vi "Find Target Actor.vi"(5 "Target":refnum<vi>, 7 "App Inst":refnum<vi>, 8 "error in (no error)":errorcluster, 11 "Message Path":path) -> (0 "error out":errorcluster, 3 "Targeted Actor":path)   [LabVIEW 2020, in "Message Rescripter.lvlib"]
uses:
  Message Rescripter.lvlib
  <vilib>/Utility/traverseref.llb/TRef TravTarget.ctl
  <vilib>/Utility/traverseref.llb/VI Scripting - Traverse.lvlib
  <vilib>/Utility/Data Type/NI_Data Type.lvlib
  <vilib>/ErrorRing/Error Ring.xnode
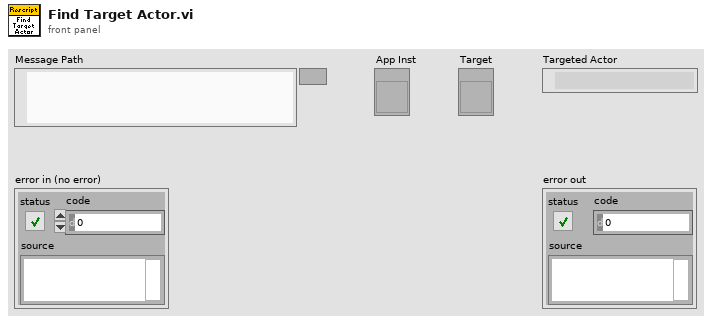
[diagram p1: front panel]
types:
  T1 = typedef "TRef TravTarget.ctl" = enum16{"FP", "BD", "Other"}
  T2 = typedef "NI_FileType.lvlib/LVFileType.ctl" = enum32{"Invalid file", "Unknown type", "Instrument", "Control", "Polymorphic VI", "Project", "Library", "LVClass", "XControl", "XNode", "Shared library", ".NET assembly", "ActiveX interface", "CIN", "Run-time menu", "Palette menu", "Help file", "LLB", "XNode Edit Dependency", "Class Private Data Control", "Statechart", "MathScript .m file", "Ladder Diagram", "LVLibp", "XNode Build Dependency"}
  T3 = cluster{"path":path, "delimited name":string, "type":T2, "iState":u32, "iStyle":u16, "wStyle":u16, "buttons":u16, "viflags":u32, "viflags2":u32, "links":u32[]}[]
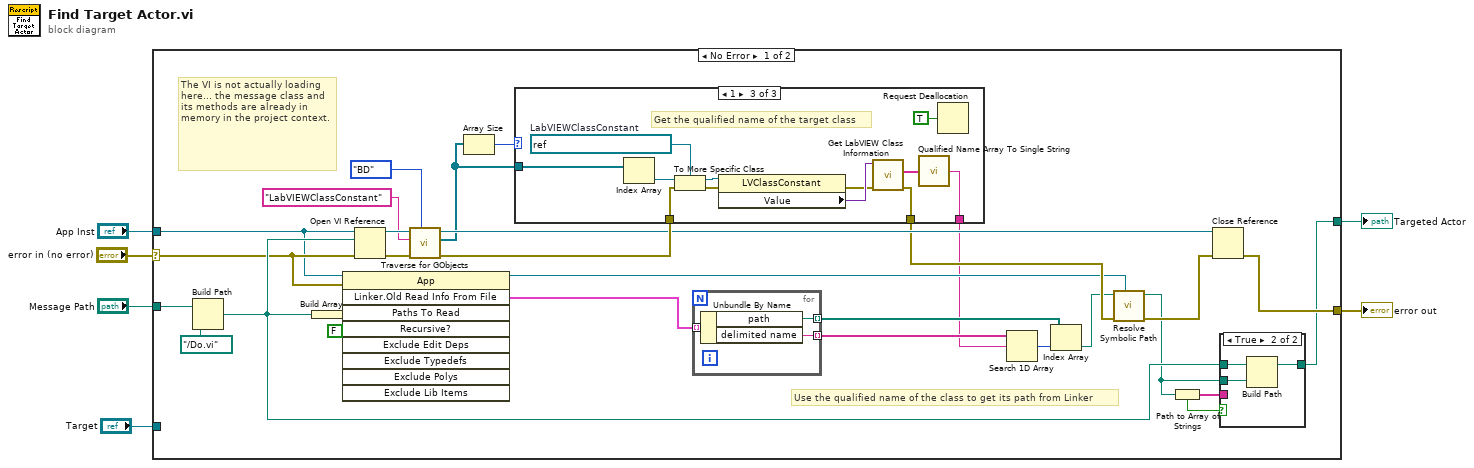
[diagram p0: block diagram]
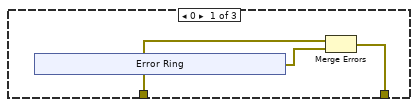
[diagram p2: hidden frame]
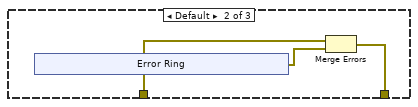
[diagram p3: hidden frame]
diagram:
  n1 = case shown="No Error" "error in (no error)" {
    selector: "error in (no error)" -> [w32 w63]
    tunnel: "Message Path" -> [w35 _]
    tunnel: [w7 _] -> w5
    tunnel: "App Inst" -> [w11 _]
    tunnel: [w31 w63] -> w3
    tunnel: "Target" -> [_ _]
    frame No Error {
      # "Use the qualified name of the class to get its path from Linker"
      # "The VI is not actually loading here... the message class and its methods are already in memory in the project context."
      n2 = Build Path(base path=w35, name or relative path=path "../Do.vi") -> (appended path=w33:path)
      n3 = Build Array(w33) -> (w20:path[])
      n4 = invoke class="App" method="Linker.Old Read Info From File"(reference=w11, error in=w32, "Paths To Read"=w20, "Recursive?"=FALSE) -> (reference out=w17:refnum<vi>, "Linker.Read Info From File"=w24:T3)  [unwired: 5 in, 7 out]
      n5 = Open VI Reference(application reference (local)=w11, vi path=w33, error in (no error)=w32) -> (vi reference=w30:refnum<vi>, error out=w29:errorcluster)  [unwired: 3 in]
      n6 = call <vilib>:"Traverse for GObjects.vi"("Traverse Target"=TRef_TravTarget."BD", "error in (no error)"=w29, "Class Name"="LabVIEWClassConstant", "VI Refnum"=w30) -> ("error out"=w26:errorcluster, "References"=w10:refnum<vi>[], "dup VI Refnum"=w25:refnum<vi>)  [unwired: 4 in, 1 out]
      n7 = Array Size(array=w10) -> (size(s)=w9:i32)
      n8 = case shown="1" w9 {
        tunnel: w26 -> [w38 w42 w53]
        tunnel: [w37 w41 w48] -> w18
        tunnel: [_ _ w46] -> w8
        tunnel: w10 -> [_ _ w44]
        frame 0 {
          n9 = xnode "Error Ring"() -> ("error out"=w36:errorcluster)
          n10 = Merge Errors(w38, w36) -> (w37:errorcluster)
        }
        frame Default {
          n11 = xnode "Error Ring"() -> ("error out"=w40:errorcluster)
          n12 = Merge Errors(w42, w40) -> (w41:errorcluster)
        }
        frame 1 {
          w55 = refnum<vi> refnum  # LabVIEWClassConstant
          # "Get the qualified name of the target class"
          n13 = Index Array(array=w44) -> (element=w51:refnum<vi>)  [unwired: 1 in]
          n14 = To More Specific Class(target class=w55, reference=w51, error in=w53) -> (specific class reference=w54:refnum<vi>, error out=w52:errorcluster)
          n15 = property class="LVClassConstant"(reference=w54, error in=w52) -> (error out=w49:errorcluster, "Value"=w50:variant)  [unwired: 1 out]
          n16 = call <vilib>:"Get LabVIEW Class Information.vi"("error in (no error)"=w49, "variant"=w50) -> ("error out"=w48:errorcluster, "qualified LabVIEW class name"=w47:string[])  [unwired: 7 in, 1 out]
          n17 = call <vilib>:"Qualified Name Array To Single String.vi"("Fully Qualified Array"=w47) -> ("Fully Qualified String"=w46:string)
          n18 = Request Deallocation(TRUE ("flag")) -> ()
        }
      }
      n19 = for {
        tunnel: w24 -> [w58] mode=indexing
        tunnel: [w57] -> w23 mode=indexing
        tunnel: [w56] -> w21 mode=indexing
        n20 = Unbundle By Name(w58) -> ("path"=w56:path, "delimited name"=w57:string)
      }
      n21 = Search 1D Array(1D array=w23, element=w8) -> (index of element=w22:i32)  [unwired: 1 in]
      n22 = Index Array(array=w21, index=w22) -> (element=w16:path)
      n23 = call "Resolve Symbolic Path.vi"("App Inst"=w17, "error in (no error)"=w18, "Path"=w16) -> ("error out"=w15:errorcluster, "Resolved Path"=w12:path)  [unwired: 7 in]
      n24 = Path to Array of Strings(0:w12) -> (1:w13:bool, 2:w14:string[])
      n25 = Close Reference(reference=w25, error in (no error)=w15) -> (error out=w31:errorcluster)
      n26 = case shown="True" w13 {
        tunnel: w12 -> [w59 w60]
        tunnel: w14 -> [_ _]
        tunnel: w33 -> [_ w62]
        tunnel: [w59 w61] -> w7
        frame False {
        }
        frame True {
          n27 = Build Path(base path=w62, name or relative path=w60) -> (appended path=w61:path)
        }
      }
    }
    frame Error {
    }
  }
  "Targeted Actor" <- w5
  "error out" <- w3
